vi "MCA_init.vi"(0 "下阈值":u16=100, 1 "设置：信号极性（正T）":bool=TRUE, 2 "上阈值":u16=200) -> ()   [LabVIEW 2014]
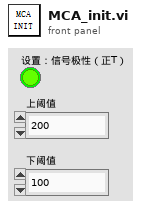
[diagram p1: front panel]
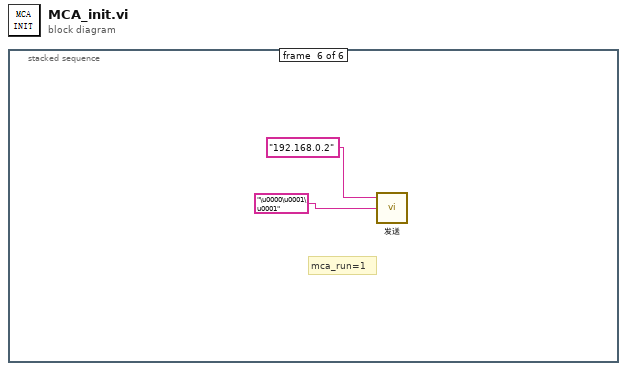
[diagram p0: block diagram]
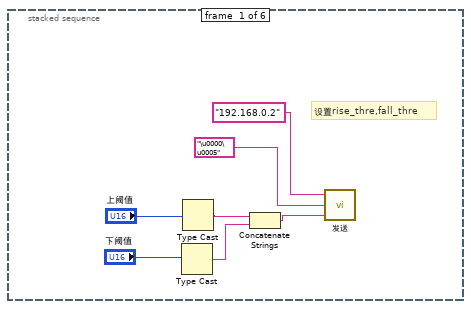
[diagram p2: hidden frame]
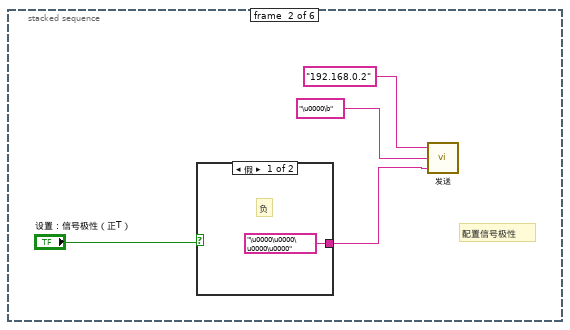
[diagram p3: hidden frame]
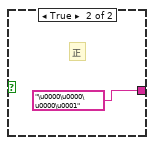
[diagram p4: hidden frame]
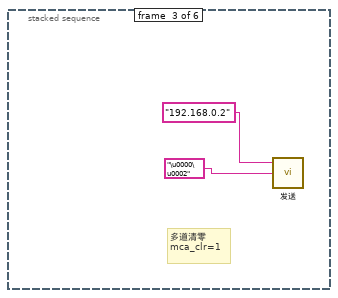
[diagram p5: hidden frame]
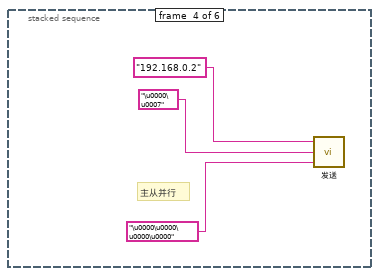
[diagram p6: hidden frame]
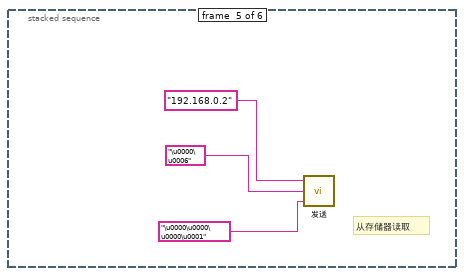
[diagram p7: hidden frame]
diagram:
  n1 = stacked-sequence {
    frame #0 {
      # "设置rise_thre,fall_thre"
      n2 = Type Cast(x="下阈值") -> (*(type *) &x=w3:string)  [unwired: 1 in]
      n3 = Type Cast(x="上阈值") -> (*(type *) &x=w6:string)  [unwired: 1 in]
      n4 = Concatenate Strings(w6, w3) -> (w4:string)
      n5 = call "发送.vi"("数据（32bit）"=w4, "命令(16bit)"="\u0000\u0005", "目标IP"="192.168.0.2") -> ()  [unwired: 1 out]
    }
    frame #1 {
      # "配置信号极性"
      n6 = case shown="假" "设置：信号极性（正T）" {
        tunnel: ["\u0000\u0000\u0000\u0000" ("数据（32bit）") "\u0000\u0000\u0000\u0001" ("数据（32bit）")] -> w9
        frame False {
          # "负"
        }
        frame True {
          # "正"
        }
      }
      n7 = call "发送.vi"("数据（32bit）"=w9, "命令(16bit)"="\u0000\b", "目标IP"="192.168.0.2") -> ()  [unwired: 1 out]
    }
    frame #2 {
      # "多道清零\nmca_clr=1"
      n8 = call "发送.vi"("命令(16bit)"="\u0000\u0002", "目标IP"="192.168.0.2") -> ()  [unwired: 1 in, 1 out]
    }
    frame #3 {
      # "主从并行"
      n9 = call "发送.vi"("数据（32bit）"="\u0000\u0000\u0000\u0000", "命令(16bit)"="\u0000\u0007", "目标IP"="192.168.0.2") -> ()  [unwired: 1 out]
    }
    frame #4 {
      # "从存储器读取"
      n10 = call "发送.vi"("数据（32bit）"="\u0000\u0000\u0000\u0001", "命令(16bit)"="\u0000\u0006", "目标IP"="192.168.0.2") -> ()  [unwired: 1 out]
    }
    frame #5 {
      # "mca_run=1"
      n11 = call "发送.vi"("命令(16bit)"="\u0000\u0001\u0001", "目标IP"="192.168.0.2") -> ()  [unwired: 1 in, 1 out]
    }
  }
